vi "LVClasse_SurfaceFloatWithPupil ctor.vi"(0 "SurfaceFloatWithPupil (const)":refnum<class "SurfaceFloatWithPupil.lvclass">, 5 "Dimensions_um":T1, 11 "error in (no error)":errorcluster) -> (4 "SurfaceFloatWithPupil (new)":refnum<class "SurfaceFloatWithPupil.lvclass">, 15 "error out":errorcluster)   [LabVIEW 2020, in "SurfaceFloatWithPupil.lvclass"]
doc: "Phase constructor from dimensions and steps.\n\n--------------------------------------------------------------------------------\n\n<B>dimensions</B> : Phase dimensions as the (width, height) of the pupil.\n<B>step</B> : Phase sampling steps in x and y direction (um).\n<B>PhaseIn</B> : Constant Pointer to Phase object.\n<B>PhaseOut</B> : Pointer to Phase object.\n<B>ErrorIn</B> : Error\n<B>ErrorOut</B> : Error\n\n--------------------------------------------------------------------------------"
uses:
  SurfaceFloatWithPupil.lvclass
  General dimensions definition.ctl
  Point2D.ctl
  Point2Df.ctl
  Handle creation.ctl
  SurfaceFloatWithPupil.lvclass/SurfaceFloatWithPupil.ctl
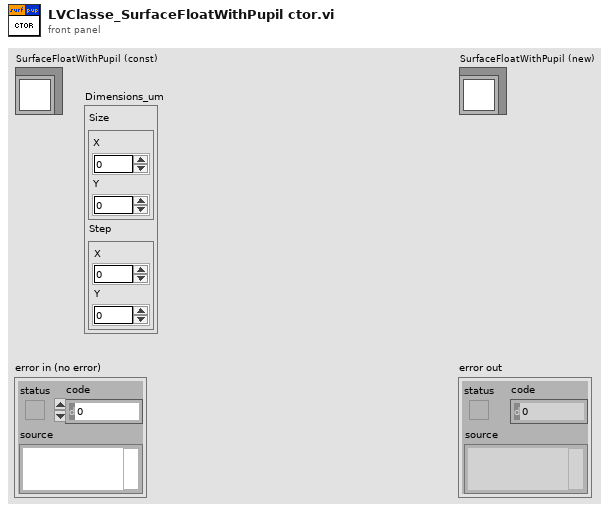
[diagram p1: front panel]
types:
  T1 = typedef "General dimensions definition.ctl" = cluster{"Size":T2, "Step":T3}
  T2 = typedef "Point2D.ctl" = cluster{"X":u32, "Y":u32}
  T3 = typedef "Point2Df.ctl" = cluster{"X":sgl, "Y":sgl}
  T4 = typedef "Handle creation.ctl" = enum16{"By ctor", "By write function"}
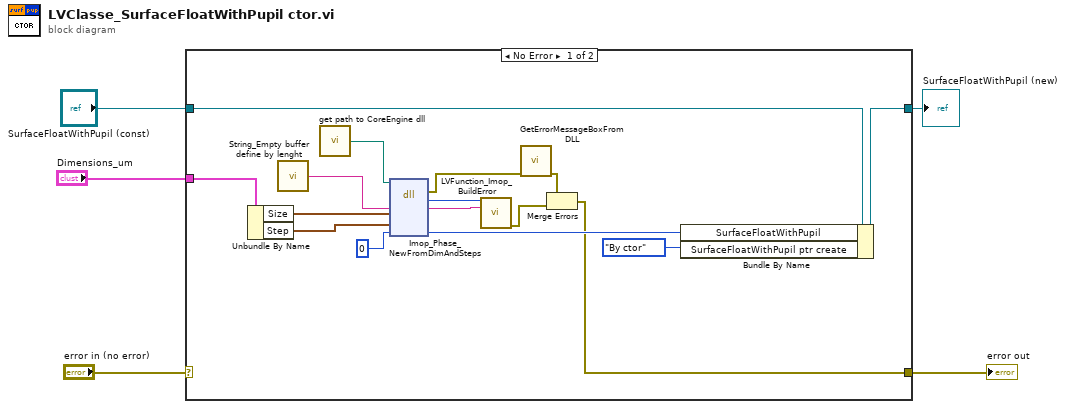
[diagram p0: block diagram]
diagram:
  n1 = case shown="No Error" "error in (no error)" {
    selector: "error in (no error)" -> [_ w23]
    tunnel: [w6 w23] -> w4
    tunnel: [w13 w22] -> w2
    tunnel: "SurfaceFloatWithPupil (const)" -> [w14 w22]
    tunnel: "Dimensions_um" -> [w12 _]
    frame No Error {
      n2 = Unbundle By Name(w12) -> ("Size"=w11:T2, "Step"=w10:T3)
      n3 = call "String_Empty buffer define by lenght.vi"() -> ("Empty buffer"=w18:string)  [unwired: 1 in]
      n4 = call "get path to CoreEngine dll.vi"() -> ("path to wavekit library"=w17:path)  [unwired: 14 in, 1 out]
      n5 = dll-call lib="D:/soft/HASO_v3/SVN_trunk/ImOpCoreEngine4_LV2011/DLLs/c_interface_vc100.dll" fn="Imop_Phase_NewFromDimAndSteps"(path in=w17, "message"=w18, "width_height"=w11, "x_step_y_step"=w10, "phase"=0 ("objet")) -> (error out=w9:errorcluster, "return type"=w21:i32, "message"=w20:string, "phase"=w19:i64)  [unwired: 4 in, 1 out]
      n6 = call "LVFunction_Imop_BuildError.vi"("code"=w21, "String to Prepend to source (\"\")"=w20) -> ("error out"=w7:errorcluster)  [unwired: 13 in]
      n7 = call "GetErrorMessageBoxFromDLL.vi"("error IN"=w9) -> ("error OUT"=w8:errorcluster)  [unwired: 10 in]
      n8 = Merge Errors(w8, w7) -> (w6:errorcluster)
      n9 = Bundle By Name(cluster=w14, "SurfaceFloatWithPupil"=w19, "SurfaceFloatWithPupil ptr create"=Handle_creation."By ctor" ("HasoData ptr create")) -> (w13:refnum<class "SurfaceFloatWithPupil.lvclass">)
    }
    frame Error {
    }
  }
  "error out" <- w4
  "SurfaceFloatWithPupil (new)" <- w2
